vi "Set Primary Destination Path.vi"(8 "error in (no error)":errorcluster, 10 "Destination path":path, 11 "Build in":refnum<class "NI_AB_API_Build.lvclass">) -> (0 "error out":errorcluster, 3 "Build out":refnum<class "NI_AB_API_Build.lvclass">)   [LabVIEW 2020, in "NI_AB_API_Build.lvclass"]
uses:
  <vilib>/AppBuilder/AB_API/Build/NI_AB_API_Build.lvclass
  <vilib>/AppBuilder/AB_API/common/AB_API Default Destinations.ctl
  <vilib>/AppBuilder/AB_API/Build/NI_AB_API_Build.lvclass/NI_AB_API_Build.ctl
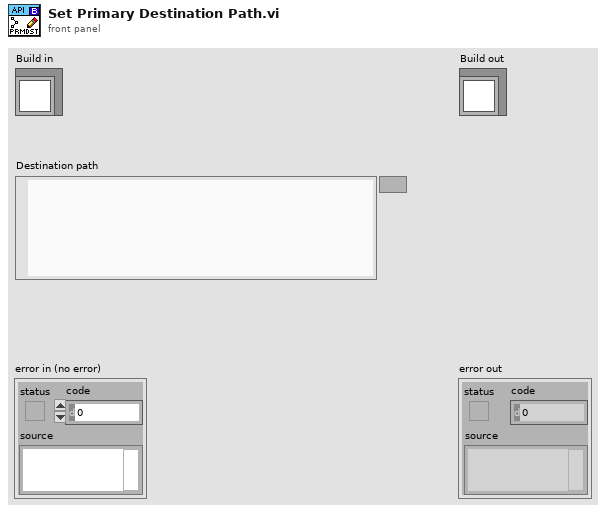
[diagram p1: front panel]
types:
  T1 = typedef "AB_API Default Destinations.ctl" = enum16{"Destination Directory", "Support Directory"}
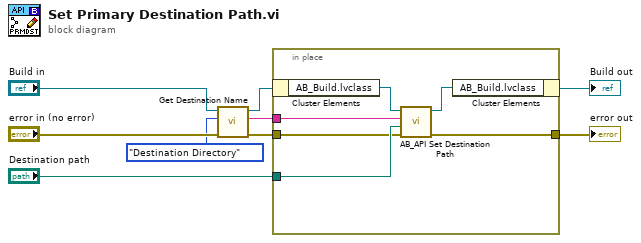
[diagram p0: block diagram]
diagram:
  n1 = call-dynamic "Get Destination Name.vi"("error in (no error)"="error in (no error)", "Default Destinations"=AB_API_Default_Destinations."Destination Directory", "NI_AB_API_Build in"="Build in") -> ("error out"=w4:errorcluster, "Destination Name"=w2:string, "NI_AB_API_Build out"=w3:refnum<class "NI_AB_API_Build.lvclass">)  [unwired: 6 in]
  n2 = in-place {
    in-place-border: w2 -> [w15]
    in-place-border: "Destination path" -> [w14]
    in-place-border: w4 -> [w13]
    in-place-border: [w12] -> w8
    n3 = in-place-cluster #1(w3) -> ("AB_Build.lvclass"=w11:refnum<class "AB_Build.lvclass">)
    n4 = call <vilib>:"AB_API Set Destination Path.vi"("error in (no error)"=w13, "Destination path"=w14, "Destination label"=w15, "Build in"=w11) -> ("error out"=w12:errorcluster, "Build out"=w10:refnum<class "AB_Build.lvclass">)  [unwired: 6 out]
    n5 = in-place-cluster #1("AB_Build.lvclass"=w10) -> (→"Build out":refnum<class "NI_AB_API_Build.lvclass">)
  }
  "error out" <- w8
